vi "Unflatten String To Variant.vi"(10 "error in (no error)":errorcluster, 11 "String":string) -> (2 "error out":errorcluster, 3 "Variant":variant)   [LabVIEW 2015, in "Utility.lvlib"]
uses:
  Utility.lvlib
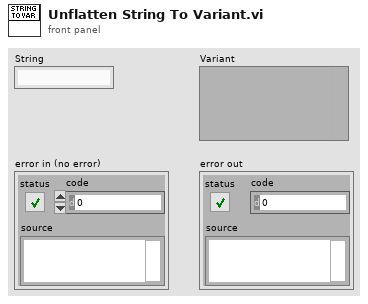
[diagram p1: front panel]
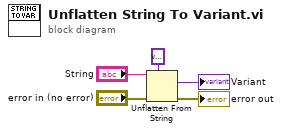
[diagram p0: block diagram]
diagram:
  n1 = Unflatten From String(type=variant, binary string="String", error in (no error)="error in (no error)") -> (value=→"Variant":variant, error out=→"error out":errorcluster)  [unwired: 2 in, 1 out]
